vi "ExecuteCommand.vi"(8 "error in (no error)":errorcluster, 10 "Command":string, 11 "VISA resource name":refnum<visa-resource-name>) -> (0 "error out":errorcluster, 2 "Response":string, 3 "VISA resource name out":refnum<visa-resource-name>)   [LabVIEW 2020, in "CAEN PSM.lvlib"]
uses:
  CAEN PSM.lvlib
  Select Event Type.ctl
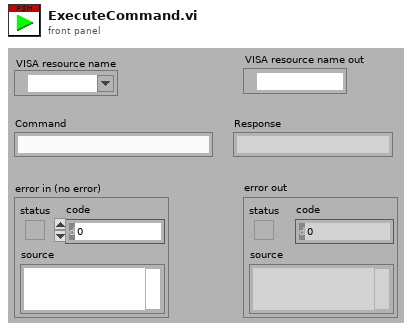
[diagram p1: front panel]
types:
  T1 = typedef "Select Event Type.ctl" = u32
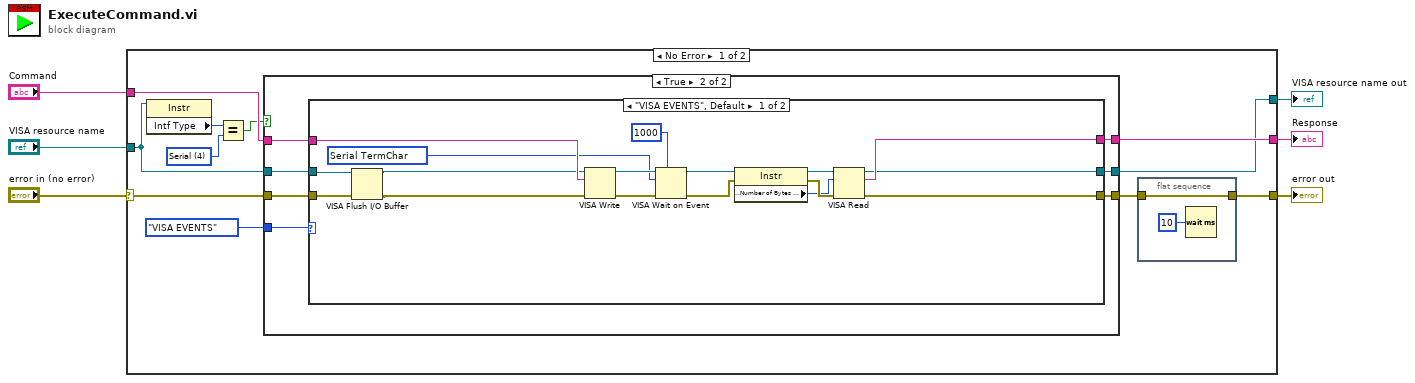
[diagram p0: block diagram]
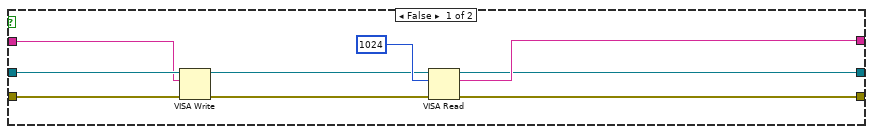
[diagram p2: hidden frame]
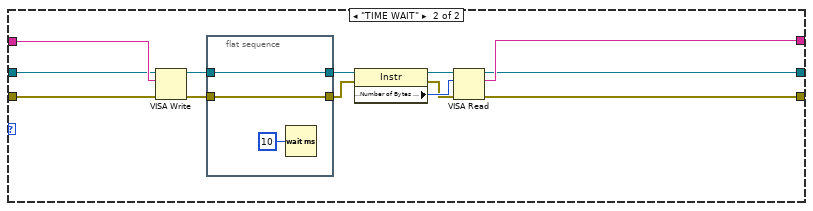
[diagram p3: hidden frame]
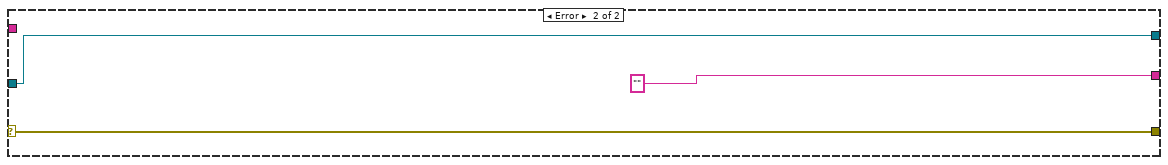
[diagram p4: hidden frame]
diagram:
  n1 = case shown="No Error" "error in (no error)" {
    selector: "error in (no error)" -> [w15 w71]
    tunnel: "Command" -> [w14 _]
    tunnel: "VISA resource name" -> [w13 w69]
    tunnel: [w17 "" ("read buffer")] -> w4
    tunnel: [w7 w71] -> w3
    tunnel: [w16 w69] -> w2
    frame No Error {
      w11 = u16 4 items=["GPIB"=1, "VXI"=2, "GPIB-VXI"=3, "Serial"=4, "PXI"=5, "TCPIP"=6, "USB"=7] ("Interface Information:Interface Type")
      n2 = property class="Instr"(reference=w13) -> ("Intf Type"=w12:u16)  [unwired: 1 in, 2 out]
      n3 = Equal?(x=w12, y=w11) -> (x = y?=w10:bool)
      n4 = case shown="True" w10 {
        tunnel: [w24 w35] -> w17
        tunnel: [w25 w31] -> w8
        tunnel: [w23 w30] -> w16
        tunnel: w13 -> [w27 w34]
        tunnel: w15 -> [w28 w33]
        tunnel: w14 -> [w21 w32]
        tunnel: enum16{"VISA EVENTS", "TIME WAIT"}."VISA EVENTS" -> [_ w29]
        frame False {
          n5 = VISA Write(VISA resource name=w27, write buffer=w21, error in (no error)=w28) -> (VISA resource name out=w20:refnum<visa-resource-name>, error out=w26:errorcluster)  [unwired: 1 out]
          n6 = VISA Read(VISA resource name=w20, byte count=u32 1024, error in (no error)=w26) -> (VISA resource name out=w23:refnum<visa-resource-name>, read buffer=w24:string, error out=w25:errorcluster)  [unwired: 1 out]
        }
        frame True {
          n7 = case shown="\"VISA EVENTS\", Default" w29 {
            tunnel: [w52 w65] -> w35
            tunnel: w34 -> [w41 w59]
            tunnel: w33 -> [w42 w60]
            tunnel: w32 -> [w48 w61]
            tunnel: [w37 w58] -> w31
            tunnel: [w36 w57] -> w30
            frame "VISA EVENTS", Default {
              w43 = T1 1073684516 items=["Service Request"=1073684491, "Trigger"=3221168138, "Clear"=1073684493, "VXI Signal"=1073684512, "VXI/VME Interrupt"=3221168161, "VXI/VME Sysfail"=1073684509, "VXI/VME Sysreset"=1073684510, "GPIB CIC"=1073684498, "GPIB Talk"=1073684499, "GPIB Listen"=1073684500, "PXI Interrupt"=1073684514, "Serial Break"=1073684515, "Serial TermChar"=1073684516, "Serial CTS"=1073684521, "Serial DSR"=1073684522, "Serial DCD"=1073684524, "Serial RI"=1073684526, "Serial Character"=1073684533, "USB Interrupt"=1073684535, "All Enabled"=1073709055] ("Event Type")
              n8 = VISA Flush I/O Buffer(VISA resource name=w41, error in (no error)=w42) -> (VISA resource name out=w39:refnum<visa-resource-name>, error out=w40:errorcluster)  [unwired: 1 in]
              n9 = VISA Write(VISA resource name=w39, write buffer=w48, error in (no error)=w40) -> (VISA resource name out=w47:refnum<visa-resource-name>, error out=w46:errorcluster)  [unwired: 1 out]
              n10 = VISA Wait on Event(7:u32 1000 ("timeout (0)"), 8:w46, 10:w43, 11:w47) -> (0:w44:errorcluster, 3:w45:refnum<visa-resource-name>)  [unwired: 1 in, 2 out]
              n11 = property class="Instr"(reference=w45, error in=w44) -> (reference out=w50:refnum<visa-resource-name>, error out=w49:errorcluster, "Serial Settings:Number of Bytes at Serial Port"=w38:u32)
              n12 = VISA Read(VISA resource name=w50, byte count=w38, error in (no error)=w49) -> (VISA resource name out=w36:refnum<visa-resource-name>, read buffer=w52:string, error out=w37:errorcluster)  [unwired: 1 out]
            }
            frame "TIME WAIT" {
              n13 = VISA Write(VISA resource name=w59, write buffer=w61, error in (no error)=w60) -> (VISA resource name out=w56:refnum<visa-resource-name>, error out=w54:errorcluster)  [unwired: 1 out]
              n14 = flat-sequence {
                tunnel: w56 -> [w68]
                tunnel: [w68] -> w55
                tunnel: w54 -> [w67]
                tunnel: [w67] -> w53
                frame #0 {
                  n15 = Wait (ms)(milliseconds to wait=u32 10) -> ()  [unwired: 1 out]
                }
              }
              n16 = property class="Instr"(reference=w55, error in=w53) -> (reference out=w63:refnum<visa-resource-name>, error out=w62:errorcluster, "Serial Settings:Number of Bytes at Serial Port"=w64:u32)
              n17 = VISA Read(VISA resource name=w63, byte count=w64, error in (no error)=w62) -> (VISA resource name out=w57:refnum<visa-resource-name>, read buffer=w65:string, error out=w58:errorcluster)  [unwired: 1 out]
            }
          }
        }
      }
      n18 = flat-sequence {
        tunnel: w8 -> [w19]
        tunnel: [w19] -> w7
        frame #0 {
          n19 = Wait (ms)(milliseconds to wait=u32 10) -> ()  [unwired: 1 out]
        }
      }
    }
    frame Error {
    }
  }
  "Response" <- w4
  "error out" <- w3
  "VISA resource name out" <- w2
